vi "Macro Dash.vi"() -> ()   [LabVIEW 2017]
panel:
  in  "Exit":bool
  in  "Tab Control":enum32{"Macro"}(tab)
  out "Boolean":bool
  out "Tank":dbl(slide) caption="Remaining Time" scale=0.0..15.0
  in  "Record Start":bool
  out "Timer":dbl format="%#.1f"
  in  "Record Stop":bool
  in  "Macro Name":string
  in  "Macro delete":bool
  in  "Macros":i32(listbox)
  # "Tab Controls allow you to have more screens."
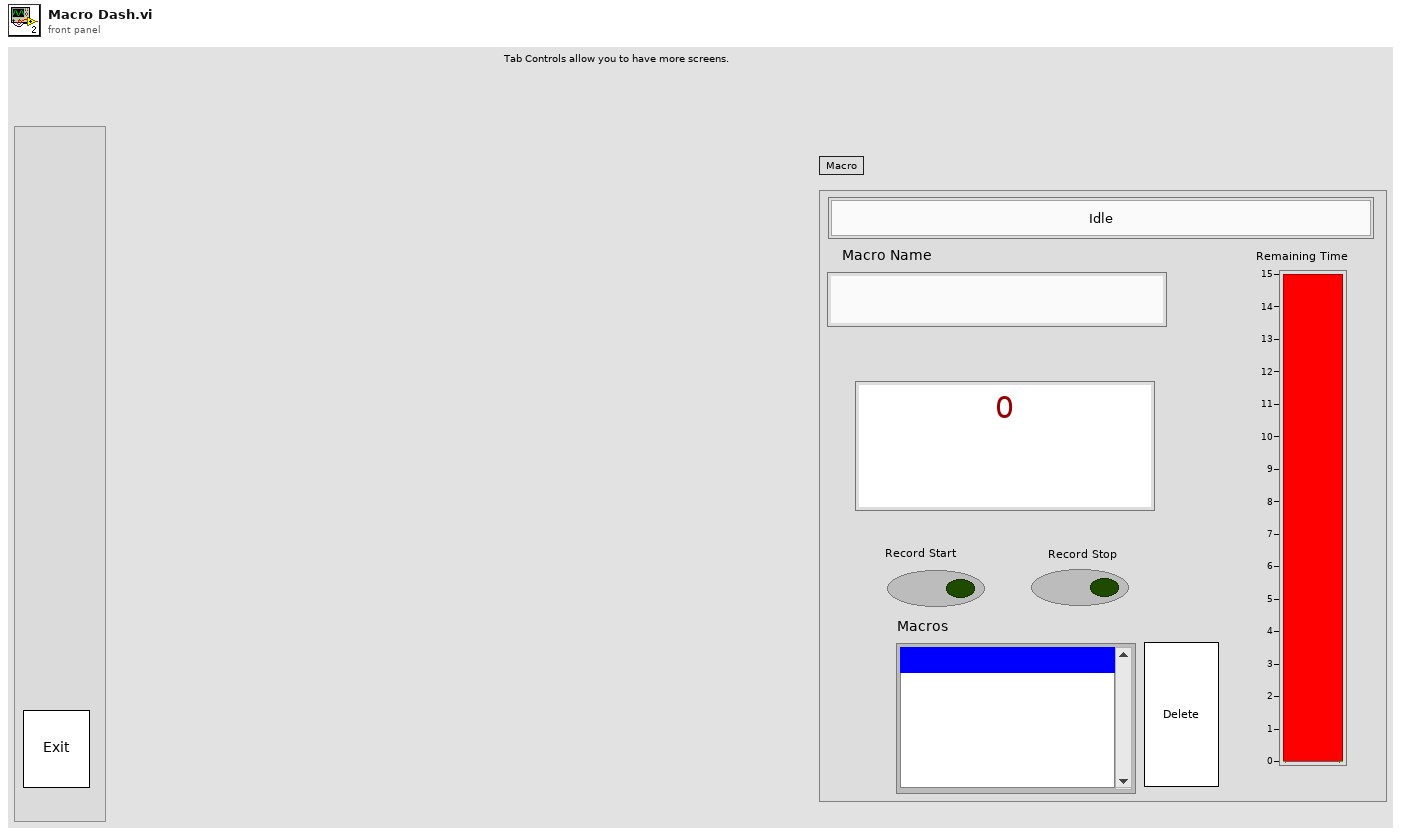
[diagram p1: front panel]
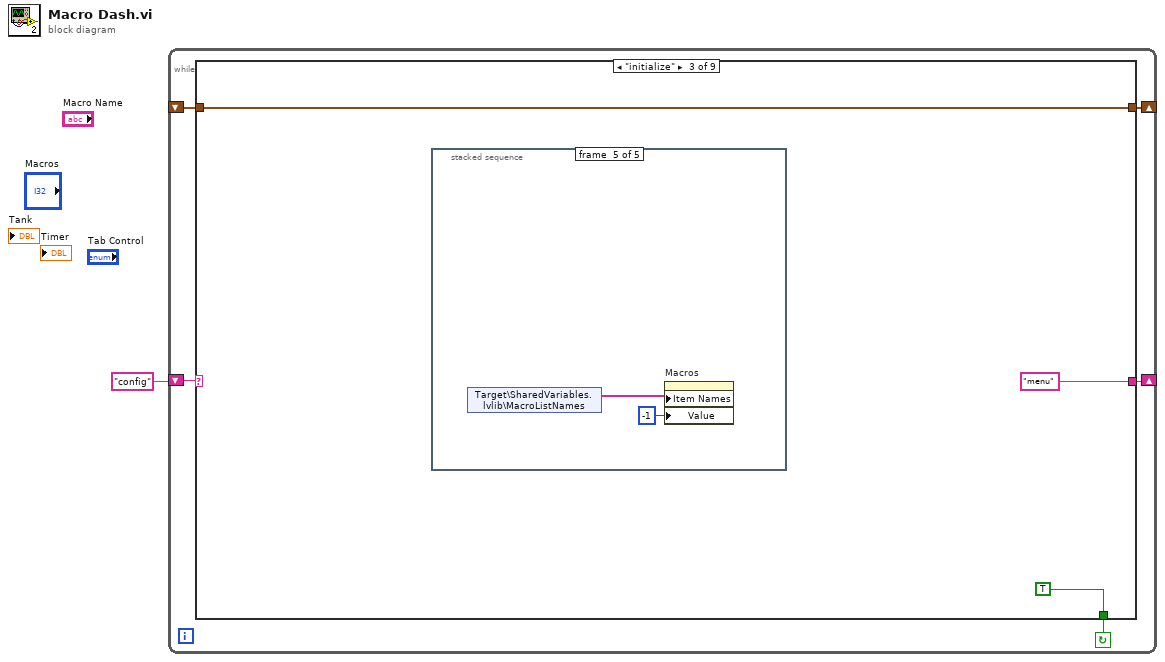
[diagram p0: block diagram]
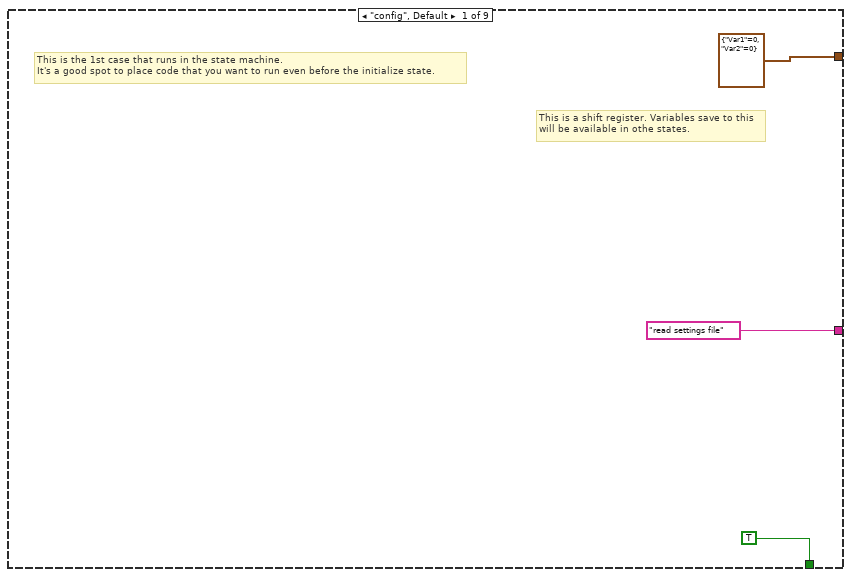
[diagram p2: hidden frame]
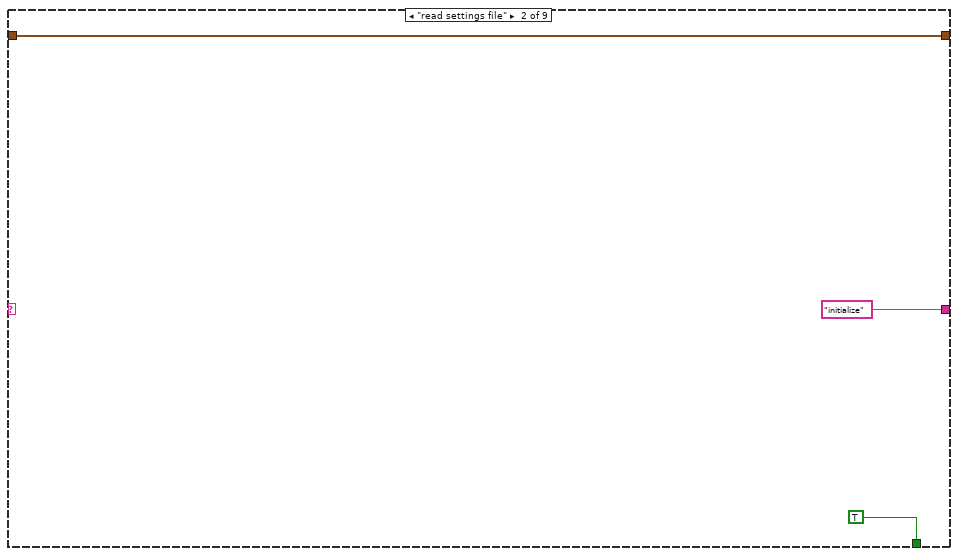
[diagram p3: hidden frame]
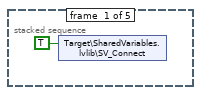
[diagram p4: hidden frame]
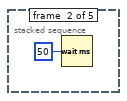
[diagram p5: hidden frame]
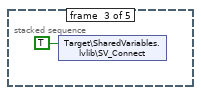
[diagram p6: hidden frame]
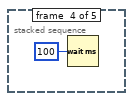
[diagram p7: hidden frame]
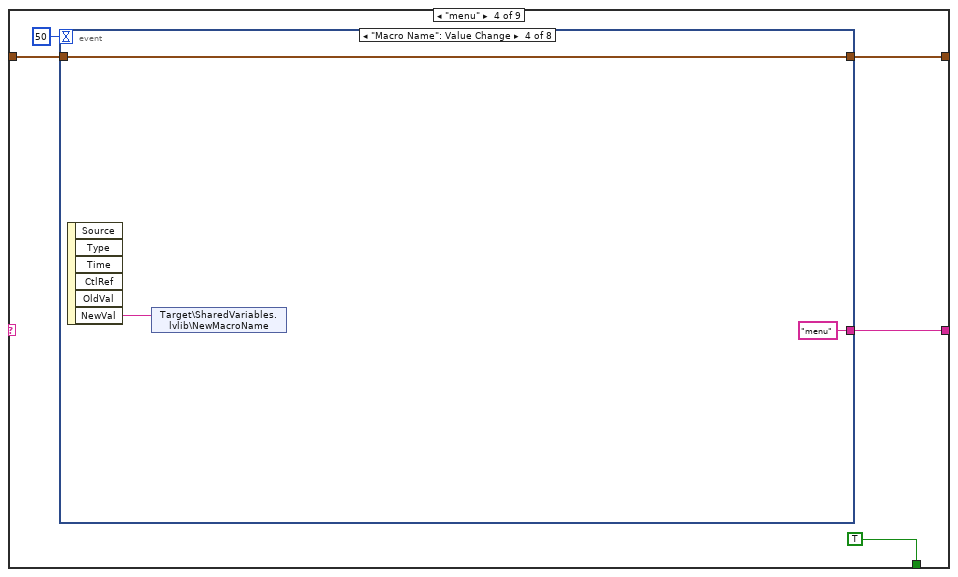
[diagram p8: hidden frame]
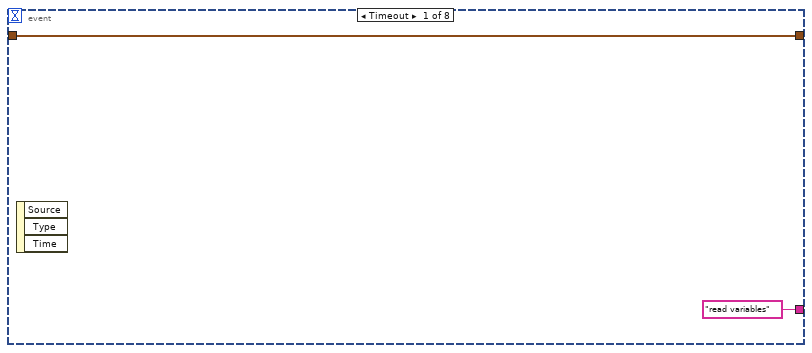
[diagram p9: hidden frame]
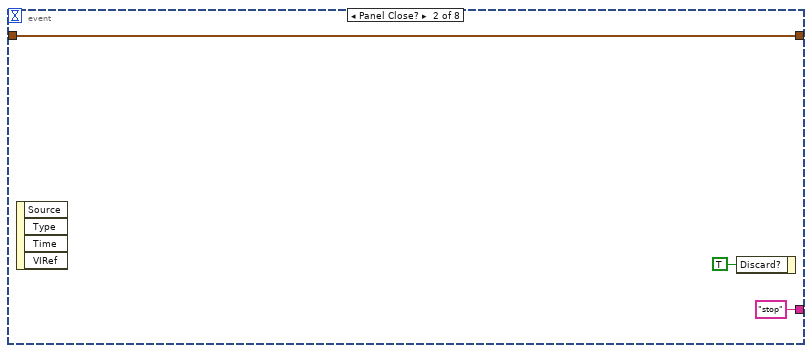
[diagram p10: hidden frame]
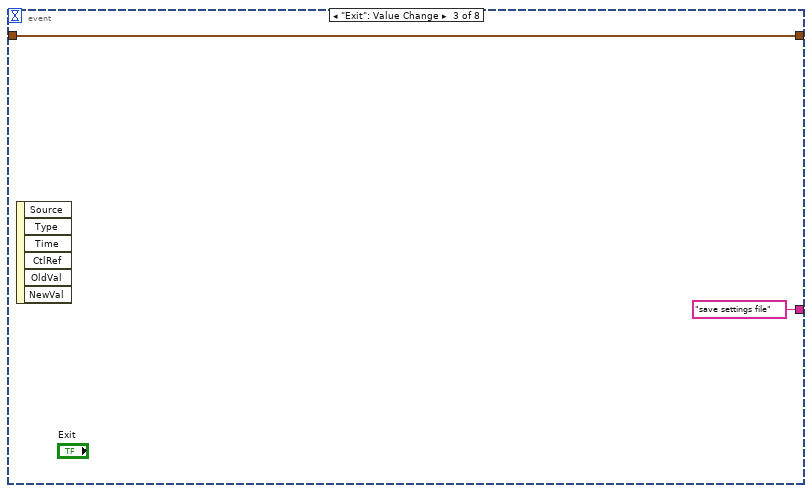
[diagram p11: hidden frame]
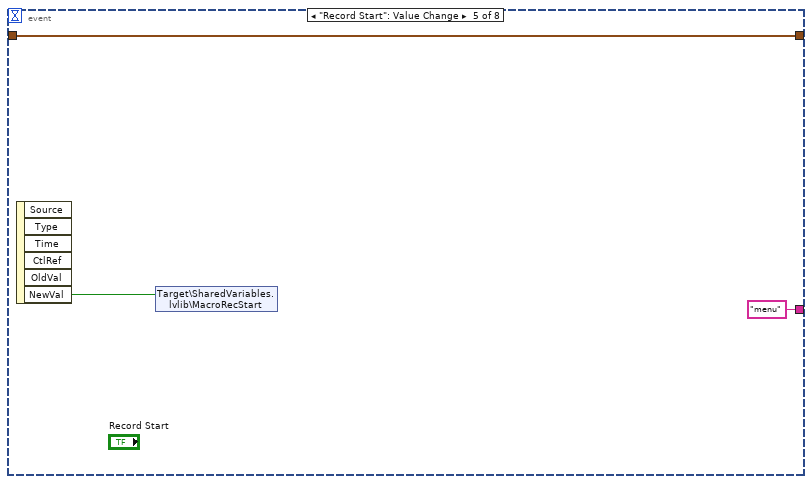
[diagram p12: hidden frame]
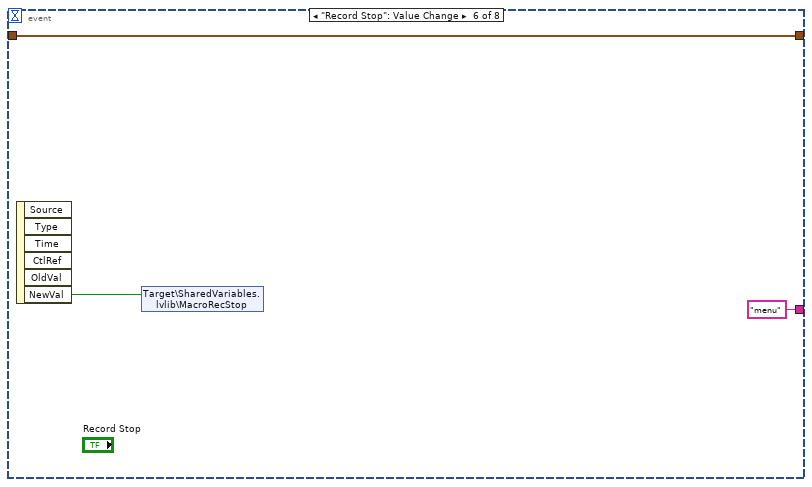
[diagram p13: hidden frame]
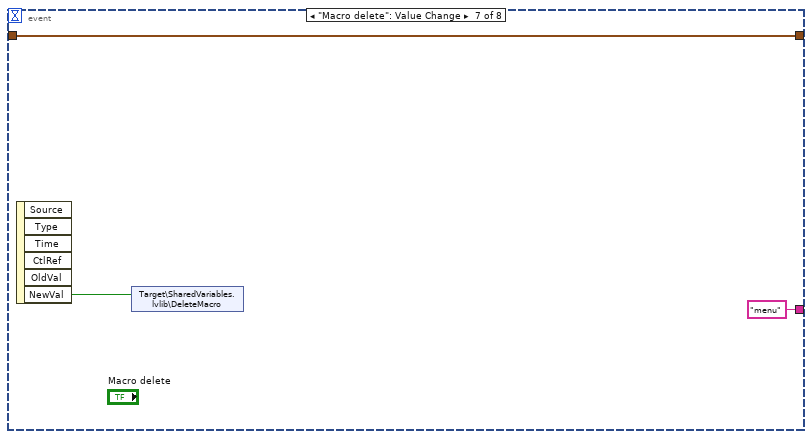
[diagram p14: hidden frame]
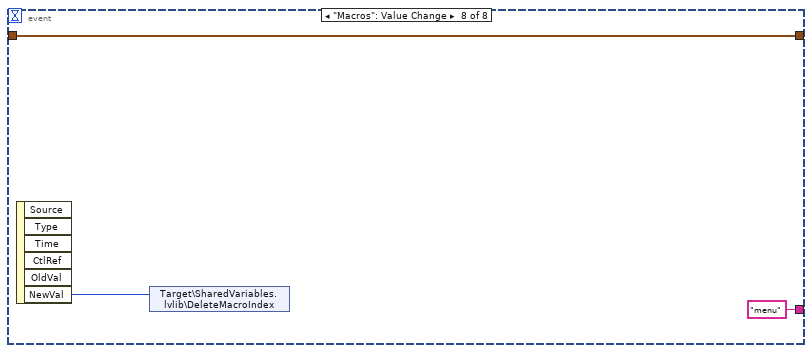
[diagram p15: hidden frame]
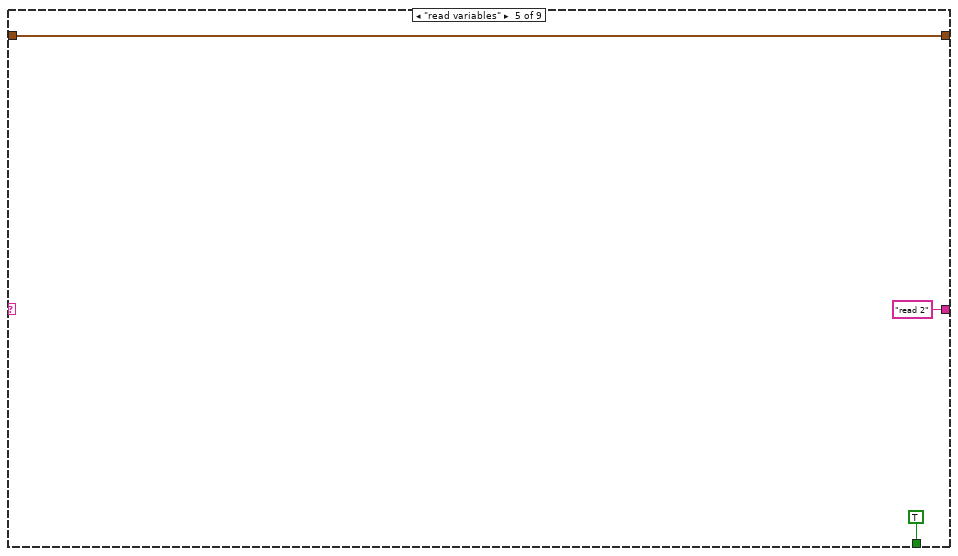
[diagram p16: hidden frame]
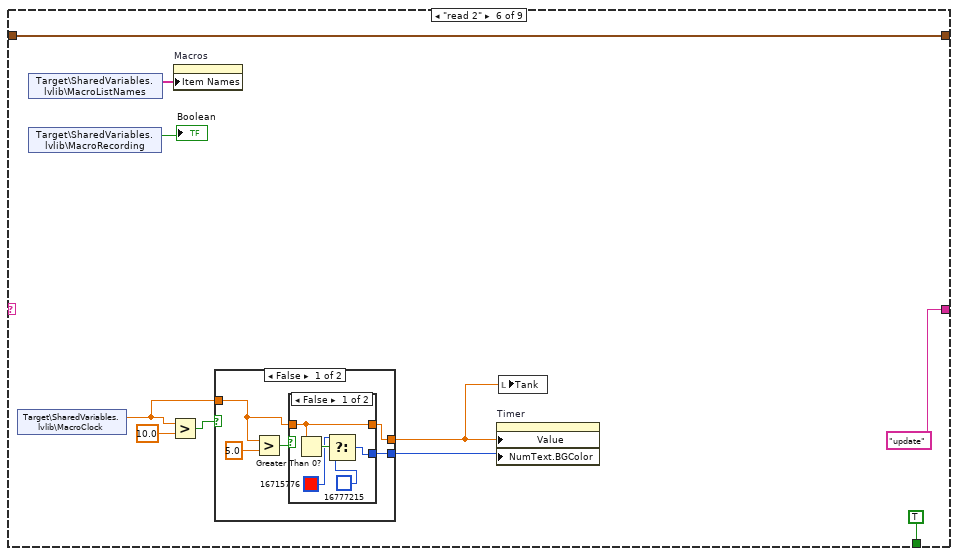
[diagram p17: hidden frame]
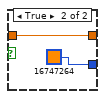
[diagram p18: hidden frame]
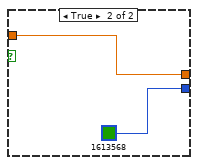
[diagram p19: hidden frame]
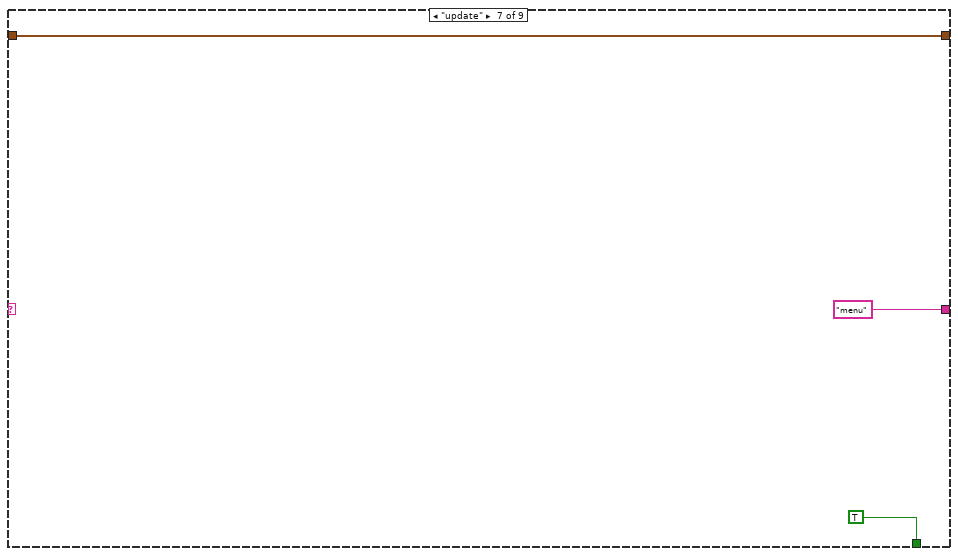
[diagram p20: hidden frame]
diagram:
  n1 = while {
    shift-right: [w4] -> _
    shift-left: "config" -> [w5]
    shift-right: [w3] -> _
    shift-left: _ -> [w2]
    stop <- w6 continue-if-true
    n2 = case shown="\"initialize\"" w5 {
      tunnel: [TRUE TRUE TRUE TRUE TRUE TRUE TRUE TRUE FALSE] -> w6
      tunnel: ["read settings file" "initialize" "menu" w25 "read 2" "update" "menu" "stop" "stop"] -> w4
      tunnel: [cluster{"Var1":i32, "Var2":i32} {"Var1"=0, "Var2"=0} w12 w13 w23 w49 w61 w78 w81 w82] -> w3
      tunnel: w2 -> [_ w12 w13 w24 w49 w61 w78 w81 w82]
      frame "config", Default {
        # "This is a shift register. Variables save to this\nwill be available in othe states."
        # "This is the 1st case that runs in the state machine.\nIt's a good spot to place code that you want to run even before the initialize state."
      }
      frame "read settings file" {
      }
      frame "initialize" {
        n3 = stacked-sequence {
          frame #0 {
            n4 = shared-variable "Target\\SharedVariables.lvlib\\SV_Connect"(TRUE ("SV_Connect")) -> ()  [unwired: 1 in, 1 out]
          }
          frame #1 {
            n5 = Wait (ms)(milliseconds to wait=u32 50) -> ()  [unwired: 1 out]
          }
          frame #2 {
            n6 = shared-variable "Target\\SharedVariables.lvlib\\SV_Connect"(TRUE ("SV_Connect")) -> ()  [unwired: 1 in, 1 out]
          }
          frame #3 {
            n7 = Wait (ms)(milliseconds to wait=u32 100) -> ()  [unwired: 1 out]
          }
          frame #4 {
            n8 = shared-variable "Target\\SharedVariables.lvlib\\MacroListNames"() -> (w21:string[])  [unwired: 1 in, 1 out]
            n9 = property on="Macros" class="LstBox (strict)"("Item Names"=w21, "Value"=-1 ("Macros")) -> ()  [unwired: 2 in, 2 out]
          }
        }
      }
      frame "menu" {
        n10 = event shown="[3] \"Macro Name\": Value Change" {
          selector: _ -> [_ _ _ _ _ _ _ _]
          dyn-events: _ -> [_ _ _ _ _ _ _ _]
          timeout: 50 -> [_ _ _ _ _ _ _ _]
          tunnel: ["read variables" "stop" "save settings file" "menu" "menu" "menu" "menu" "menu"] -> w25
          tunnel: w24 -> [w27 w31 w33 w36 w39 w42 w45 w48]
          tunnel: [w27 w31 w33 w36 w39 w42 w45 w48] -> w23
          event Timeout {
            n11 = event-data() -> ()  [unwired: 1 in, 3 out]
          }
          event Panel Close? {
            n12 = event-data() -> ()  [unwired: 1 in, 4 out]
            n13 = event-data("Discard?"=TRUE) -> ()  [unwired: 1 in, 1 out]
          }
          event "Exit": Value Change {
            n14 = event-data() -> ()  [unwired: 1 in, 6 out]
          }
          event "Macro Name": Value Change {
            n15 = event-data() -> ("NewVal"=w35:string)  [unwired: 1 in, 5 out]
            n16 = shared-variable "Target\\SharedVariables.lvlib\\NewMacroName"(w35) -> ()  [unwired: 1 in, 1 out]
          }
          event "Record Start": Value Change {
            n17 = event-data() -> ("NewVal"=w38:bool)  [unwired: 1 in, 5 out]
            n18 = shared-variable "Target\\SharedVariables.lvlib\\MacroRecStart"(w38) -> ()  [unwired: 1 in, 1 out]
          }
          event "Record Stop": Value Change {
            n19 = event-data() -> ("NewVal"=w41:bool)  [unwired: 1 in, 5 out]
            n20 = shared-variable "Target\\SharedVariables.lvlib\\MacroRecStop"(w41) -> ()  [unwired: 1 in, 1 out]
          }
          event "Macro delete": Value Change {
            n21 = event-data() -> ("NewVal"=w44:bool)  [unwired: 1 in, 5 out]
            n22 = shared-variable "Target\\SharedVariables.lvlib\\DeleteMacro"(w44) -> ()  [unwired: 1 in, 1 out]
          }
          event "Macros": Value Change {
            n23 = event-data() -> ("NewVal"=w47:i32)  [unwired: 1 in, 5 out]
            n24 = shared-variable "Target\\SharedVariables.lvlib\\DeleteMacroIndex"(w47) -> ()  [unwired: 1 in, 1 out]
          }
        }
      }
      frame "read variables" {
      }
      frame "read 2" {
        n25 = shared-variable "Target\\SharedVariables.lvlib\\MacroClock"() -> (w54:dbl)  [unwired: 1 in, 1 out]
        n26 = shared-variable "Target\\SharedVariables.lvlib\\MacroListNames"() -> (w58:string[])  [unwired: 1 in, 1 out]
        n27 = shared-variable "Target\\SharedVariables.lvlib\\MacroRecording"() -> (→"Boolean":bool)  [unwired: 1 in, 1 out]
        n28 = Greater?(x=w54, y=10.0) -> (0:w56:bool)
        n29 = property on="Macros" class="LstBox (strict)"("Item Names"=w58) -> ()  [unwired: 2 in, 2 out]
        n30 = case shown="False" w56 {
          tunnel: [w64 u32 1613568] -> w55
          tunnel: w54 -> [w63 w74]
          tunnel: [w62 w74] -> w52
          frame False {
            n31 = Greater?(x=w63, y=5.0) -> (0:w65:bool)
            n32 = case shown="False" w65 {
              tunnel: [w67 u32 16747264] -> w64
              tunnel: w63 -> [w71 w72]
              tunnel: [w71 w72] -> w62
              frame False {
                n33 = Greater Than 0?(x=w71) -> (x > 0?=w70:bool)
                n34 = Select(t=u32 16715776, s=w70, f=u32 16777215) -> (s? t:f=w67:u32)
              }
              frame True {
              }
            }
          }
          frame True {
          }
        }
        n35 = property on="Timer" class="DigNum (strict)"("Value"=w52, "NumText.BGColor"=w55) -> ()  [unwired: 2 in, 2 out]
        n36 = local write "Tank"(w52) -> ()
      }
      frame "update" {
      }
      frame "save settings file" {
      }
      frame "stop" {
        n37 = stacked-sequence {
          frame #0 {
            n38 = shared-variable "Target\\SharedVariables.lvlib\\SV_Connect"(FALSE ("SV_Connect")) -> ()  [unwired: 1 in, 1 out]
          }
          frame #1 {
            n39 = Wait (ms)(milliseconds to wait=u32 50) -> ()  [unwired: 1 out]
          }
          frame #2 {
            n40 = shared-variable "Target\\SharedVariables.lvlib\\SV_Connect"(FALSE ("SV_Connect")) -> ()  [unwired: 1 in, 1 out]
          }
          frame #3 {
            # "Only set this to TRUE when making and executable. Otherwise it will close LabVIEW."
            n41 = Quit LabVIEW(quit? (T)=FALSE) -> ()
          }
        }
      }
    }
  }
